vi "OldDemo.vi"() -> ()   [LabVIEW 2022 SP3]
uses:
  ReadOnshapeAngle.vi
  WriteOnshapeAngle.vi
panel:
  out "Angle1 Out":dbl
  out "Angle2 Out":dbl
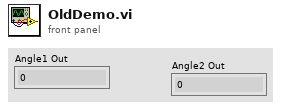
[diagram p1: front panel]
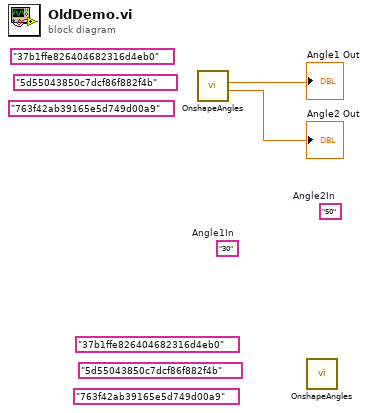
[diagram p0: block diagram]
diagram:
  (unwired) "50"  # Angle2In
  (unwired) "763f42ab39165e5d749d00a9" ("eid")
  (unwired) "5d55043850c7dcf86f882f4b" ("wid")
  (unwired) "37b1ffe826404682316d4eb0" ("did")
  (unwired) "30"  # Angle1In
  (unwired) "763f42ab39165e5d749d00a9" ("eid")
  (unwired) "5d55043850c7dcf86f882f4b" ("wid")
  (unwired) "37b1ffe826404682316d4eb0" ("did")
  n1 = call-poly "OnshapeAngles.vi"() -> ("Angle2Out"=→"Angle2 Out":dbl, "Angle1Out"=→"Angle1 Out":dbl)  [unwired: 7 in, 3 out]
  n2 = call-poly "OnshapeAngles.vi"() -> ()  [unwired: 11 in, 1 out]
